vi "LVTestInit.vi"() -> ()   [LabVIEW 2018]
uses:
  milGrabber/vs2017/x64/Debug/milGrabberInterface.dll
panel:
  out "error out":errorcluster
  out "int":i32
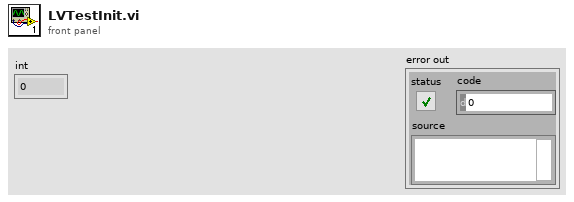
[diagram p1: front panel]
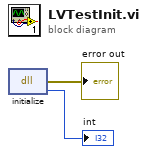
[diagram p0: block diagram]
diagram:
  n1 = dll-call lib="C:/Users/Kinga/Desktop/Matrox/Testy/milGrabber/vs2017/x64/Debug/milGrabberInterface.dll" fn="initialize"() -> (error out=→"error out":errorcluster, "int"=→"int":i32)  [unwired: 3 in, 1 out]
